vi "Exemple_Metrics_Silhouette_Samples.vi"() -> ()   [LabVIEW 2020]
uses:
  Objet/3 - Model selection and evaluation/3.3 - Metrics and scoring/silhouette_samples/Silhouette_Samples.vi
panel:
  out "Data":T1
  out "error out":errorcluster caption="sortie d'erreur"
  in  "silhouette_samples":cluster{"metric":string}={"metric"="euclidean"}
  in  "error in (no error)":errorcluster caption="entrée d'erreur (pas d'erreur)"
  in  "labels":string[][](array[string])=[["1"], ["1"], ["2"], ["4"], ["3"]]
  in  "X":string[][](array[string])=[["1", "6"], ["2", "7"], ["3", "8"], ["4", "9"], ["5", "0"]]
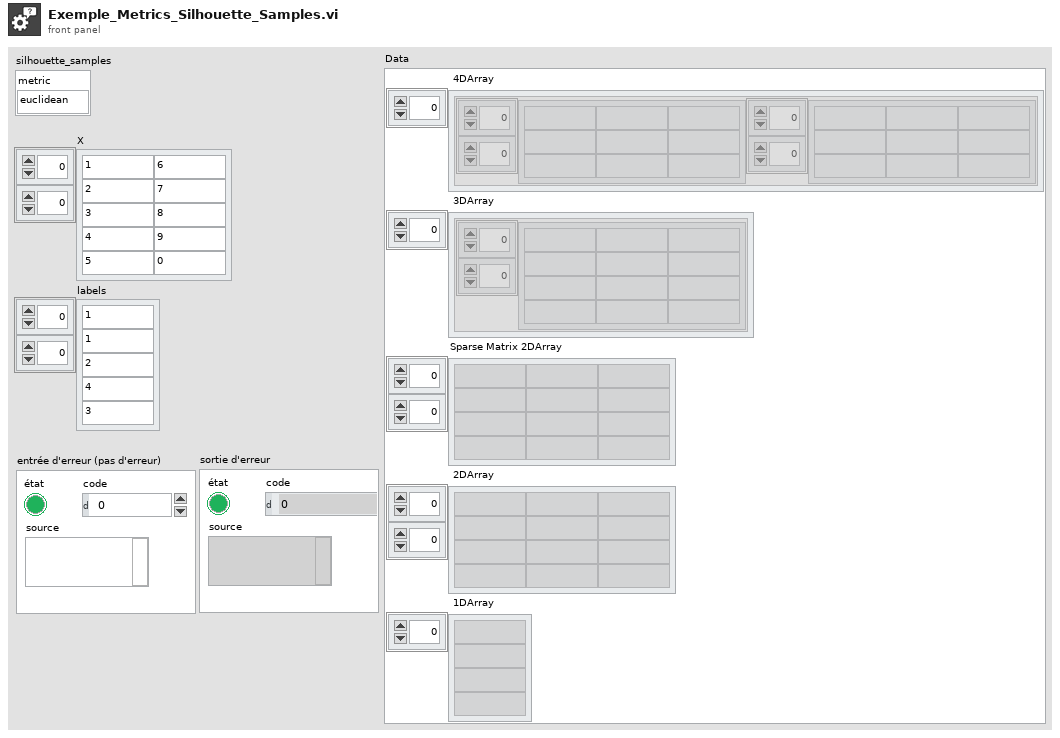
[diagram p1: front panel]
types:
  T1 = cluster{" 4DArray":cluster{"1":string[][], "2":string[][]}[], " 3DArray":cluster{"Tableau":string[][]}[], "Sparse Matrix 2DArray":string[][], " 2DArray":string[][], " 1DArray":string[]}
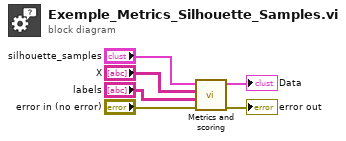
[diagram p0: block diagram]
diagram:
  n1 = call-poly "Metrics and scoring.vi"("error in (no error)"="error in (no error)", "labels"="labels", "X"="X", "silhouette_samples"="silhouette_samples") -> ("error out"=→"error out":errorcluster, "Data"=→"Data":T1)  [unwired: 6 in]
